vi "imagereg.vi"() -> ()   [LabVIEW 2012]
uses:
  <vilib>/Analysis/baseanly.llb/Mean (DBL).vi
  <vilib>/Analysis/NI_AALBase.lvlib
panel:
  in  "Tab":enum32{"Camera Init.", "Acquire"}(tab)
  in  "Constant\nfluor. amps":u16[](array[numeric])=[595, 455, 150, 360, 150]
  in  "Constant\npower amps":u16[](array[numeric])=[248, 455, 132, 266, 475]
  in  "DualView amps":u16[](array[numeric])=[1023, 760, 260, 800, 10]
  out "Initialize":u32
  out "Initialize?":bool
  out "x pixels":i32
  out "y pixels":i32
  out "Bits per Channel":i32
  out "Camera ID":string="0"
  out "Model":string="0"
  out "camera initialization error":errorcluster
  in  "Path":path
  in  "Contrast\nAdjust":cluster{i32, i32}(slide) scale=100.0..65535.0
  in  "Snap and save":bool
  out "Camera error":errorcluster caption="File error"
  in  "Enter live mode":bool
  in  "Exposure (msec)":dbl=100.0 min=1.0 max=5000.0 step=1.0
  out "Image":u16[][](graph)
  in  "stop program":bool
  out "File error":errorcluster
  in  "Red":bool
  in  "Yellow":bool
  in  "Orange":bool
  in  "Green":bool
  in  "Blue":bool
  in  "All":bool
  in  "RedP":bool
  in  "OrangeP":bool
  in  "GreenP":bool
  in  "YellowP":bool
  in  "BlueP":bool
  in  "rEff":dbl=0.99915395 format="%#_3g"
  in  "oEff":dbl=0.99914441 format="%#_3g"
  in  "yEff":dbl=0.99909989 format="%#_3g"
  in  "gEff":dbl=0.9990684 format="%#_3g"
  in  "bEff":dbl=0.99824746 format="%#_3g"
  in  "Emission filter":u16(ring)=2 items=["ET525/30"=7, "ET510LP"=1, "ET575/50"=2, "708/75"=3, "620LP"=4, "ET590/50M"=5, "HQ660LP"=6]
  out "mean":dbl=701.2764784557547
  out "max value":u16=1056
  out "min value":u16=384
  out "Histogram":T1(graph)={"X Values"=[417.6, 484.8, 552.0, 619.2, 686.4, 753.6, 820.8, 888.0, 955.2, 1022.4], "Histogram: h(x)"=[403, 4234, 6440, 8496, 9541, 10568, 10361, 4568, 669, 48]}
  in  "White Light Current (mA)":dbl=700.0
  in  "White LED":bool
  in  "Allow Manual Contrast Adj":bool
  in  "Clicky on Image":bool
  out "Output":dbl[][](array[numeric])
  # "Default AOTF settings (calibrated values are shown on the right)"
  # "595"
  # "455"
  # "150"
  # "360"
  # "150"
  # "248"
  # "455"
  # "132"
  # "266"
  # "475"
  # "700"
  # "760"
  # "260"
  # "800"
  # "40"
  # "Main Program"
  # "Live Controls"
  # "Shutter Control"
  # "AOTF Control"
  # "Laser Power Control"
  # "Measurements"
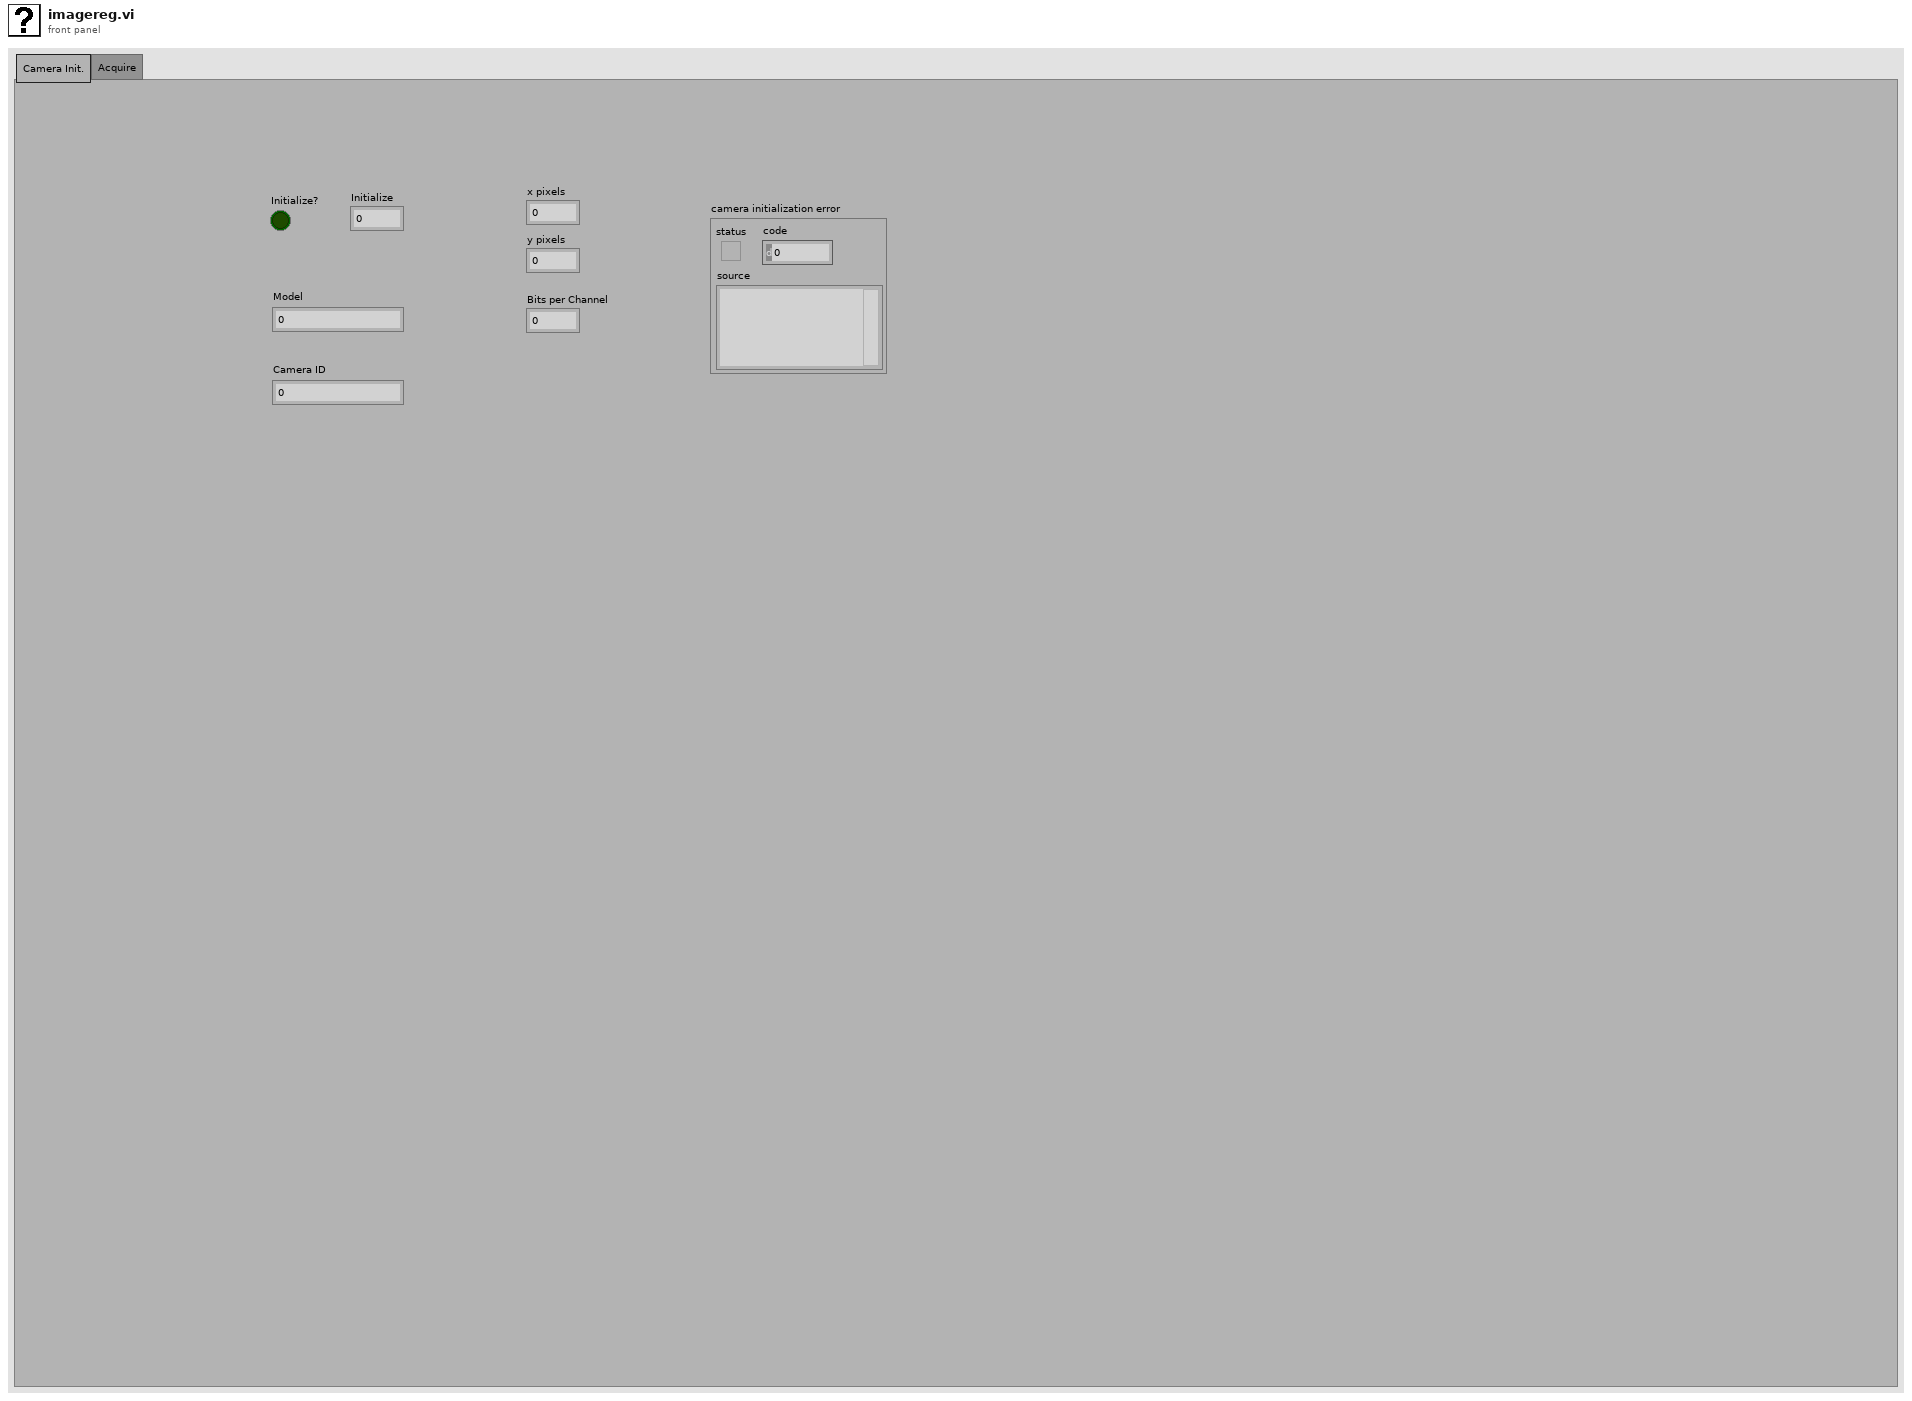
[diagram p1: front panel]
types:
  T1 = cluster{"X Values":dbl[], "Histogram: h(x)":i32[]}
  T2 = cluster{"Horizontal Offset":i32, "Vertical Offset":i32, "Horizontal Width":i32, "Vertical Width":i32}
  T3 = cluster{"Value":i32, "Minimum":i32, "Maximum":i32, "Increment":i32}
  T4 = cluster{"width":u32, "height":u32, "datatype":u32}
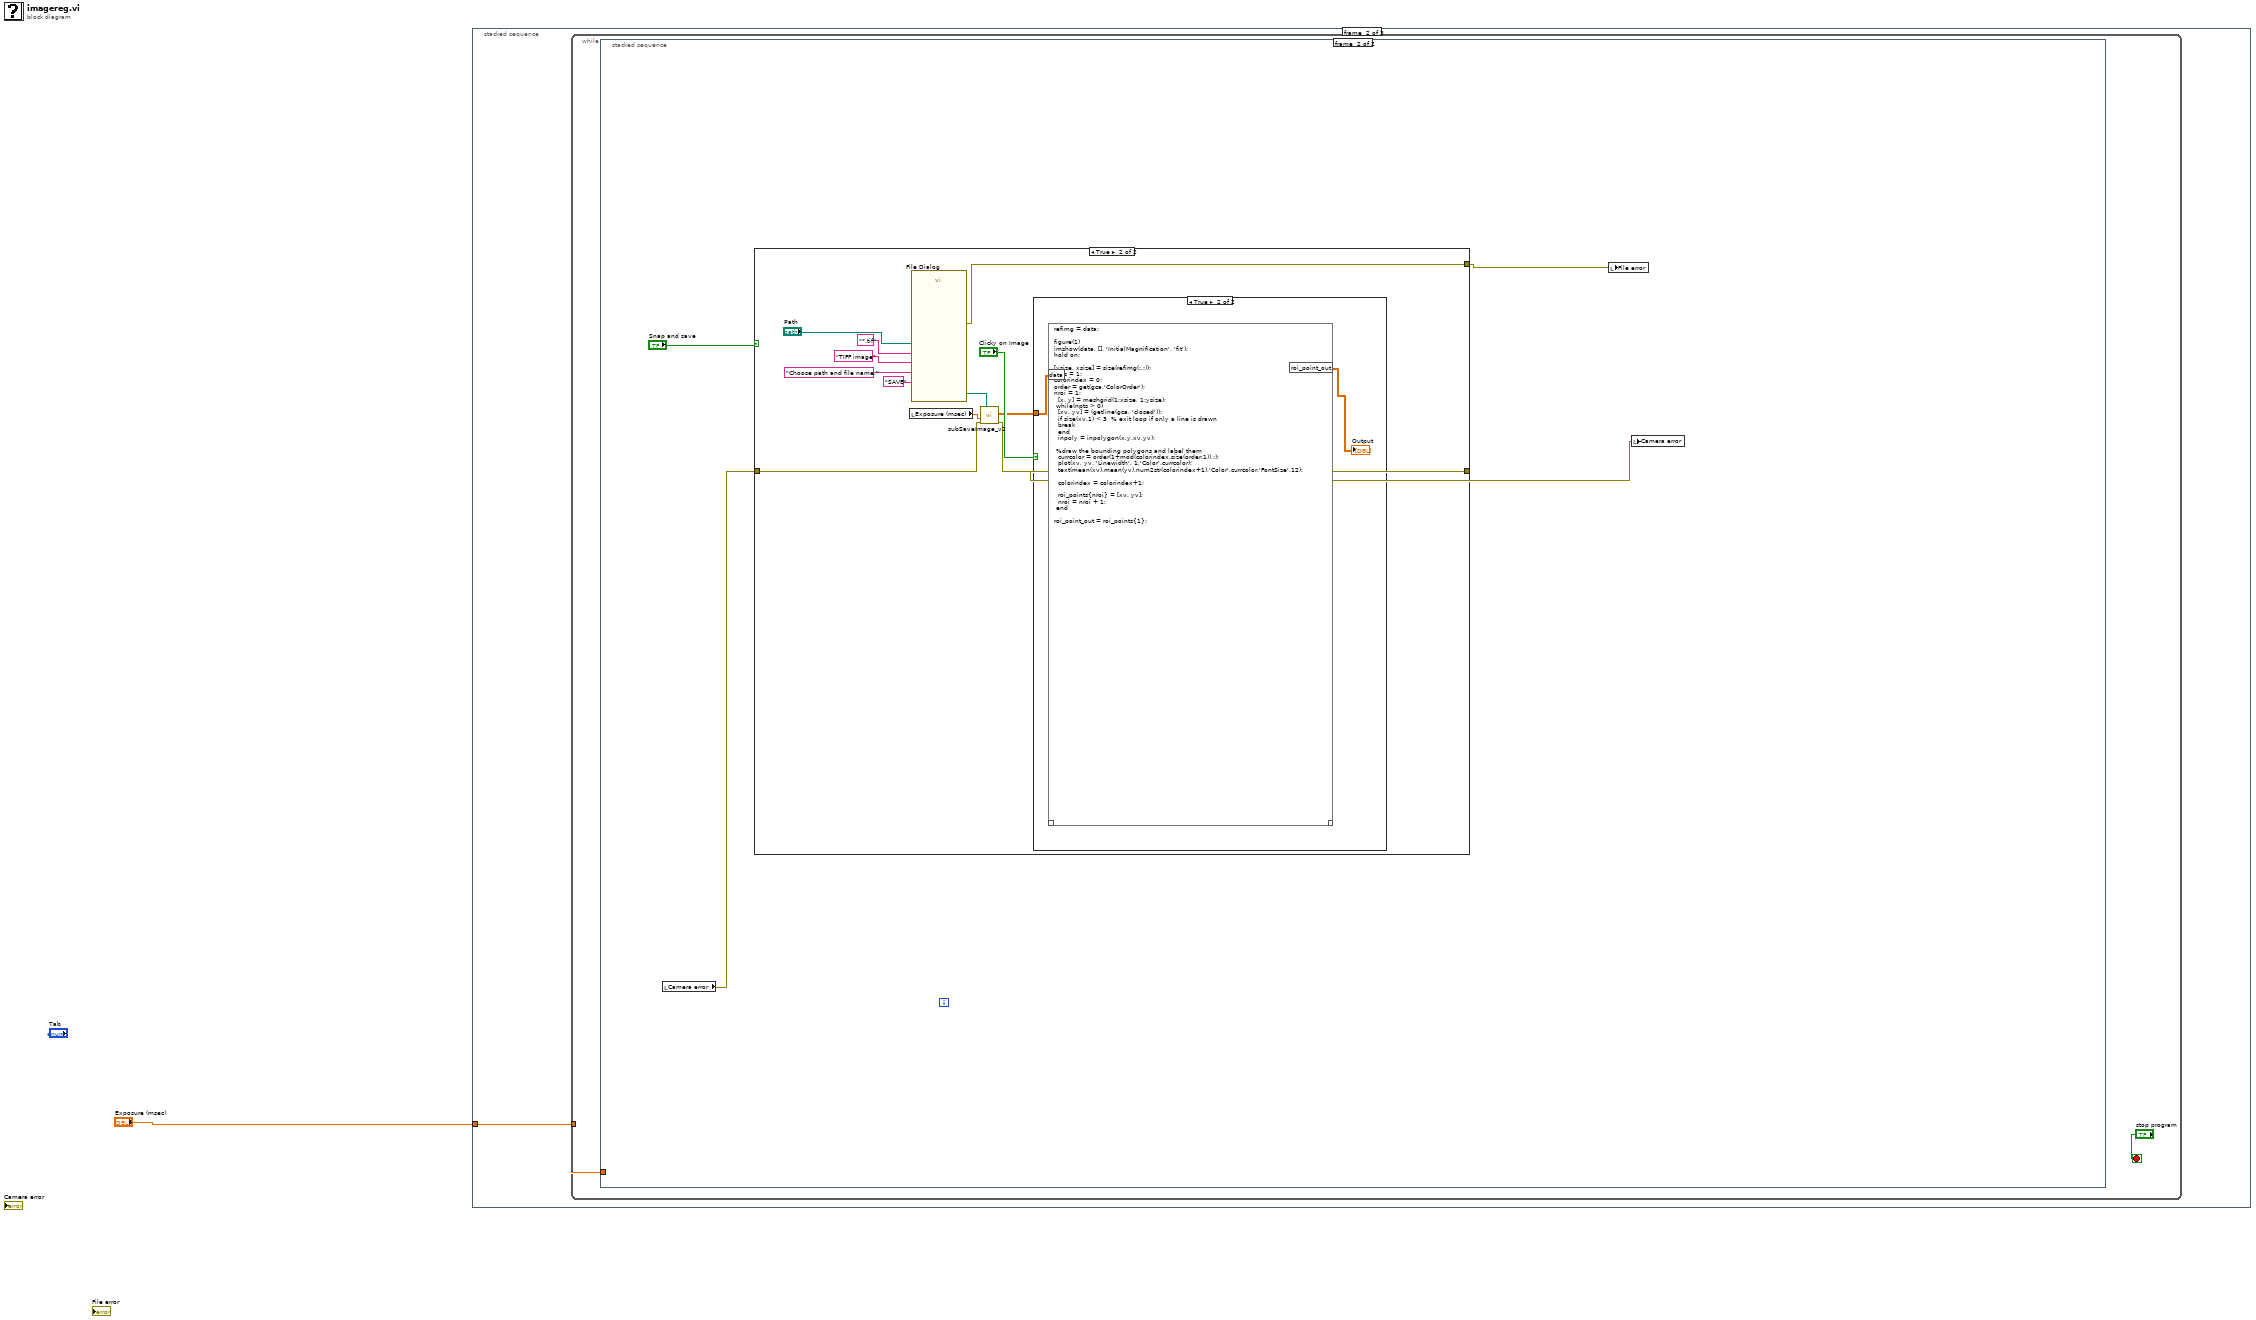
[diagram p0: block diagram]
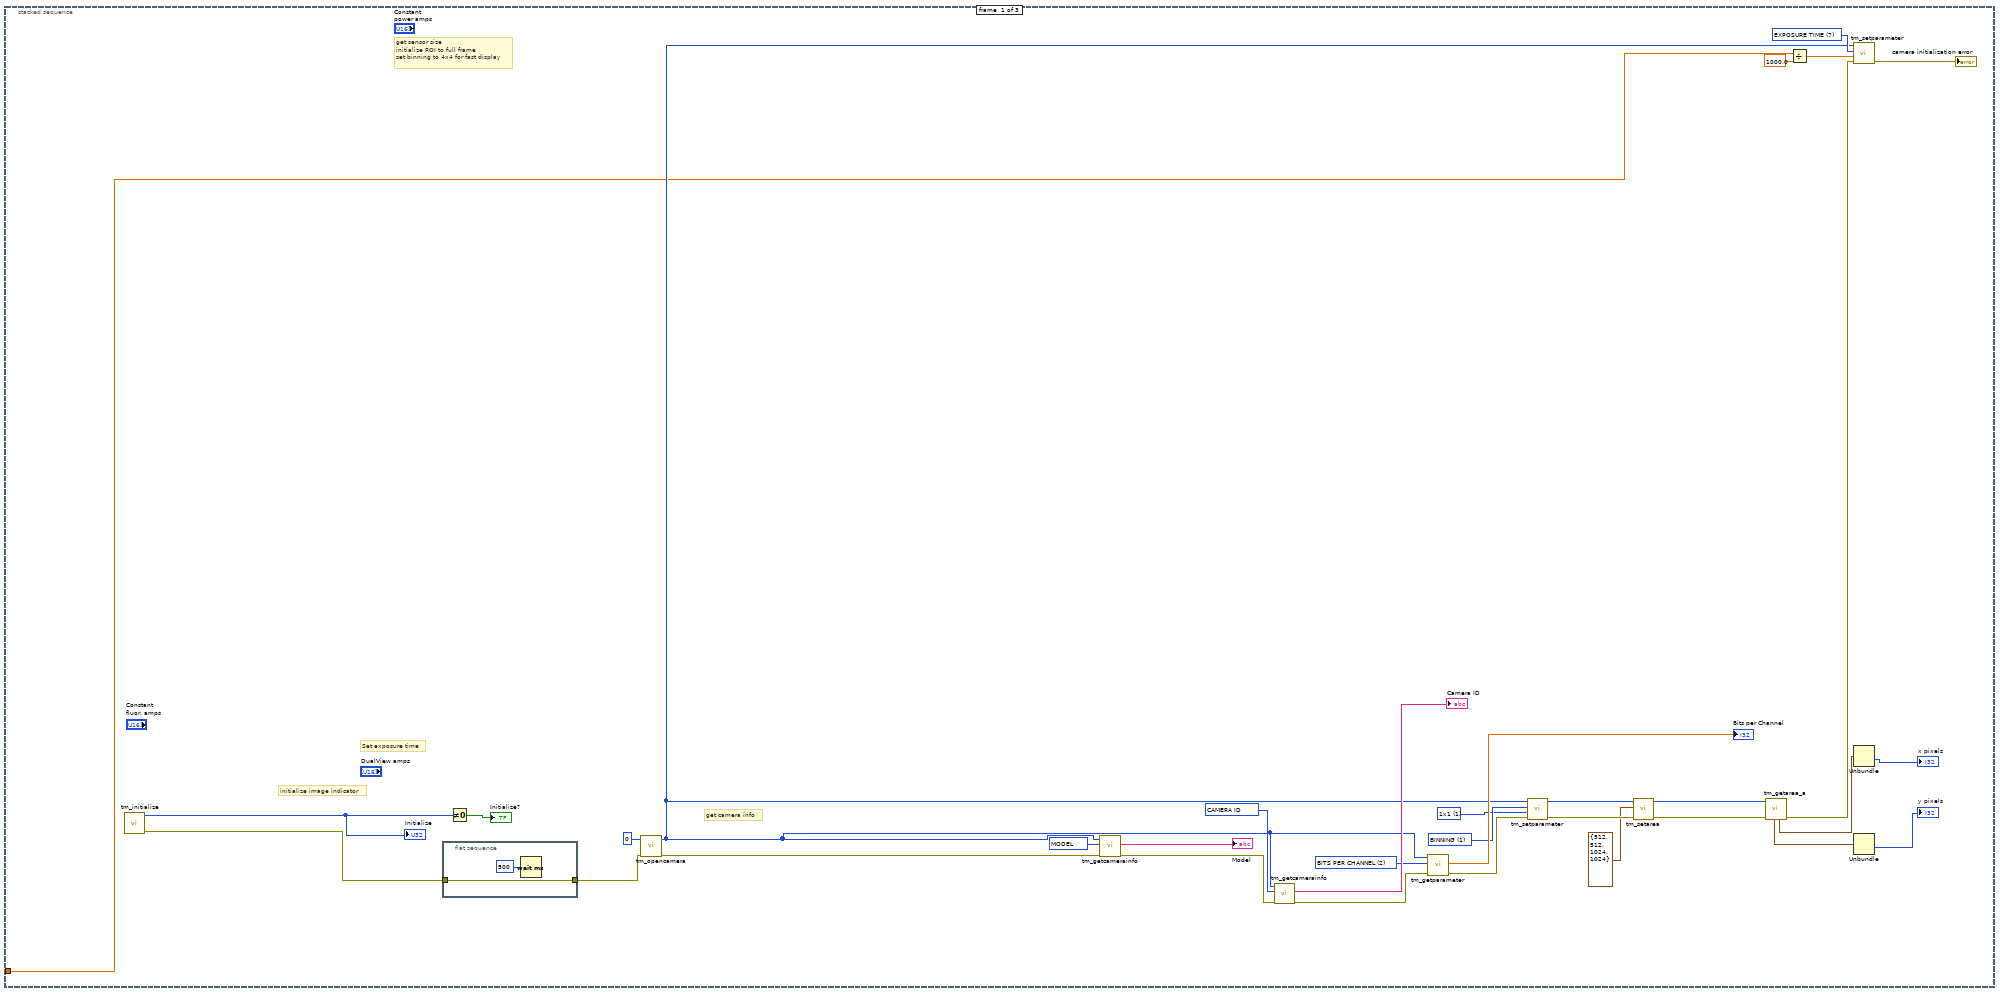
[diagram p2: hidden frame]
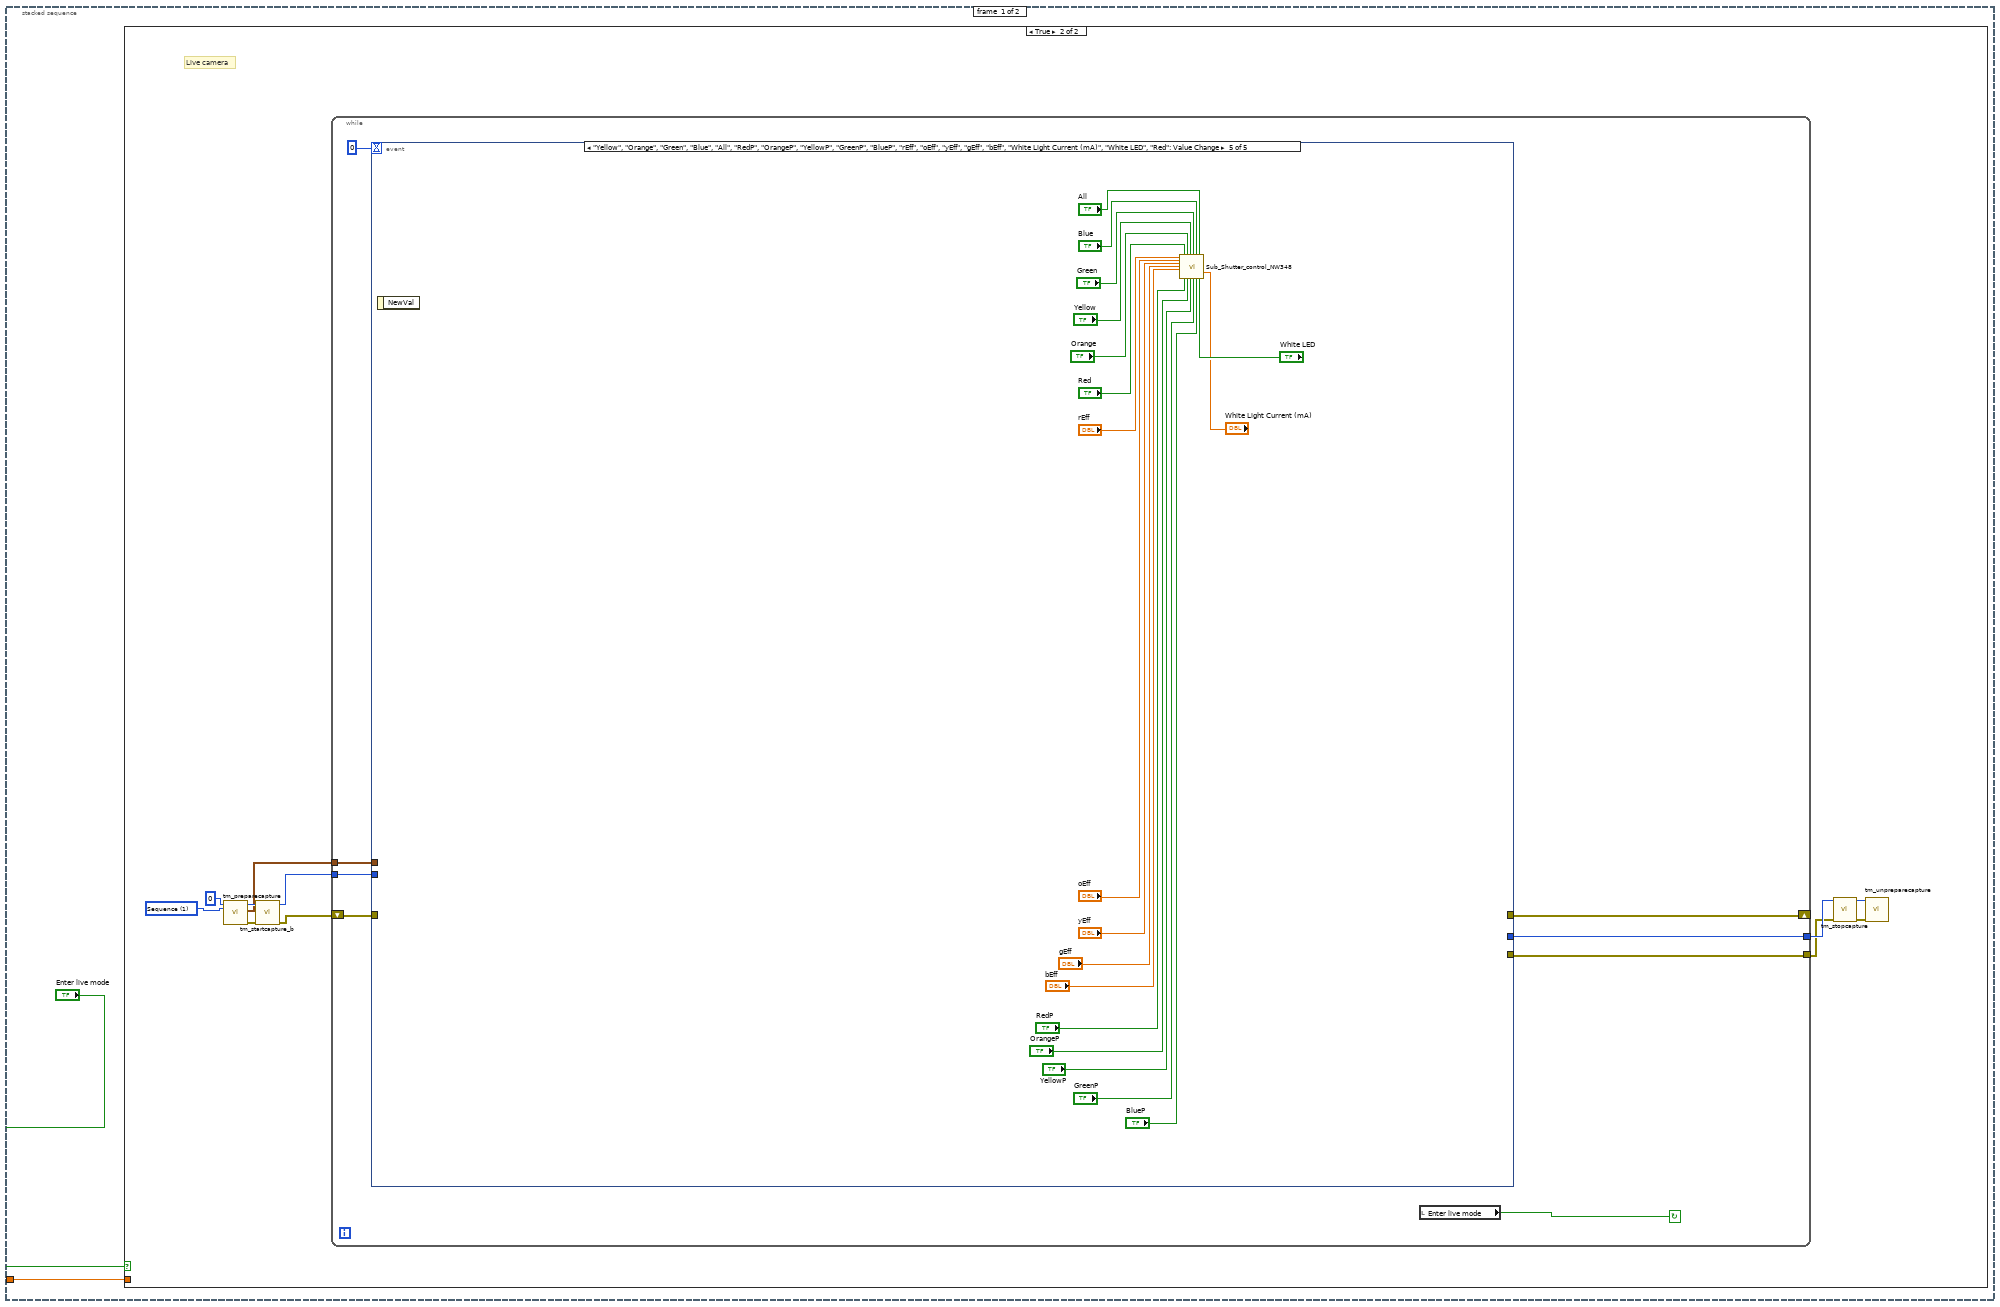
[diagram p3: hidden frame]
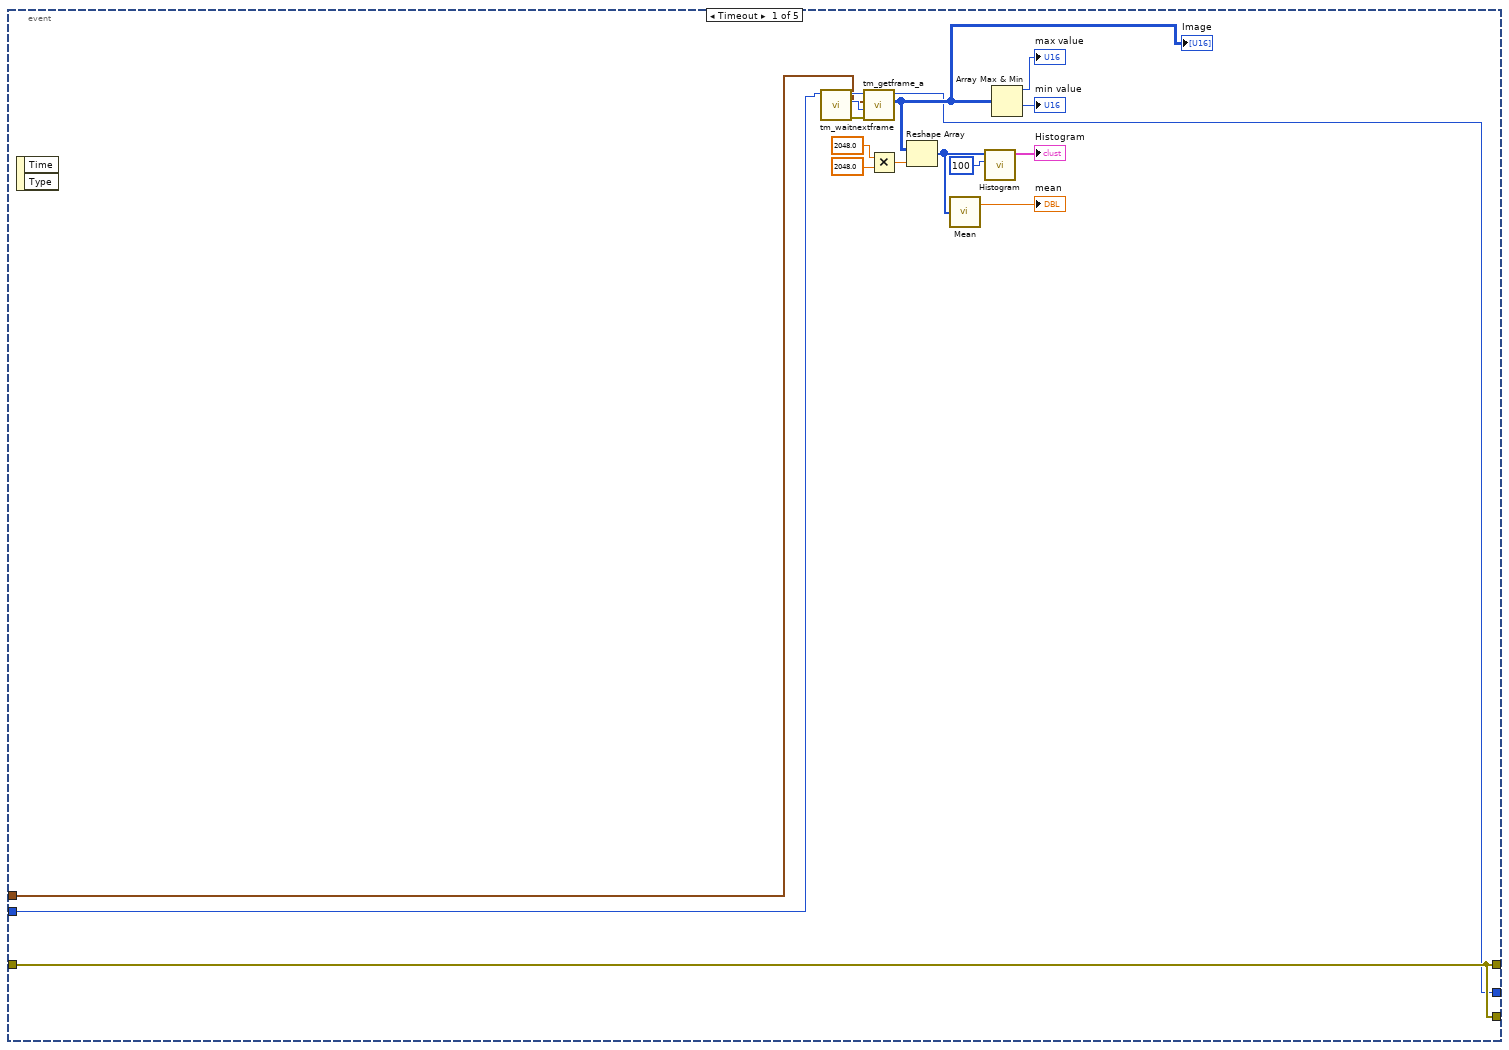
[diagram p5: hidden frame]
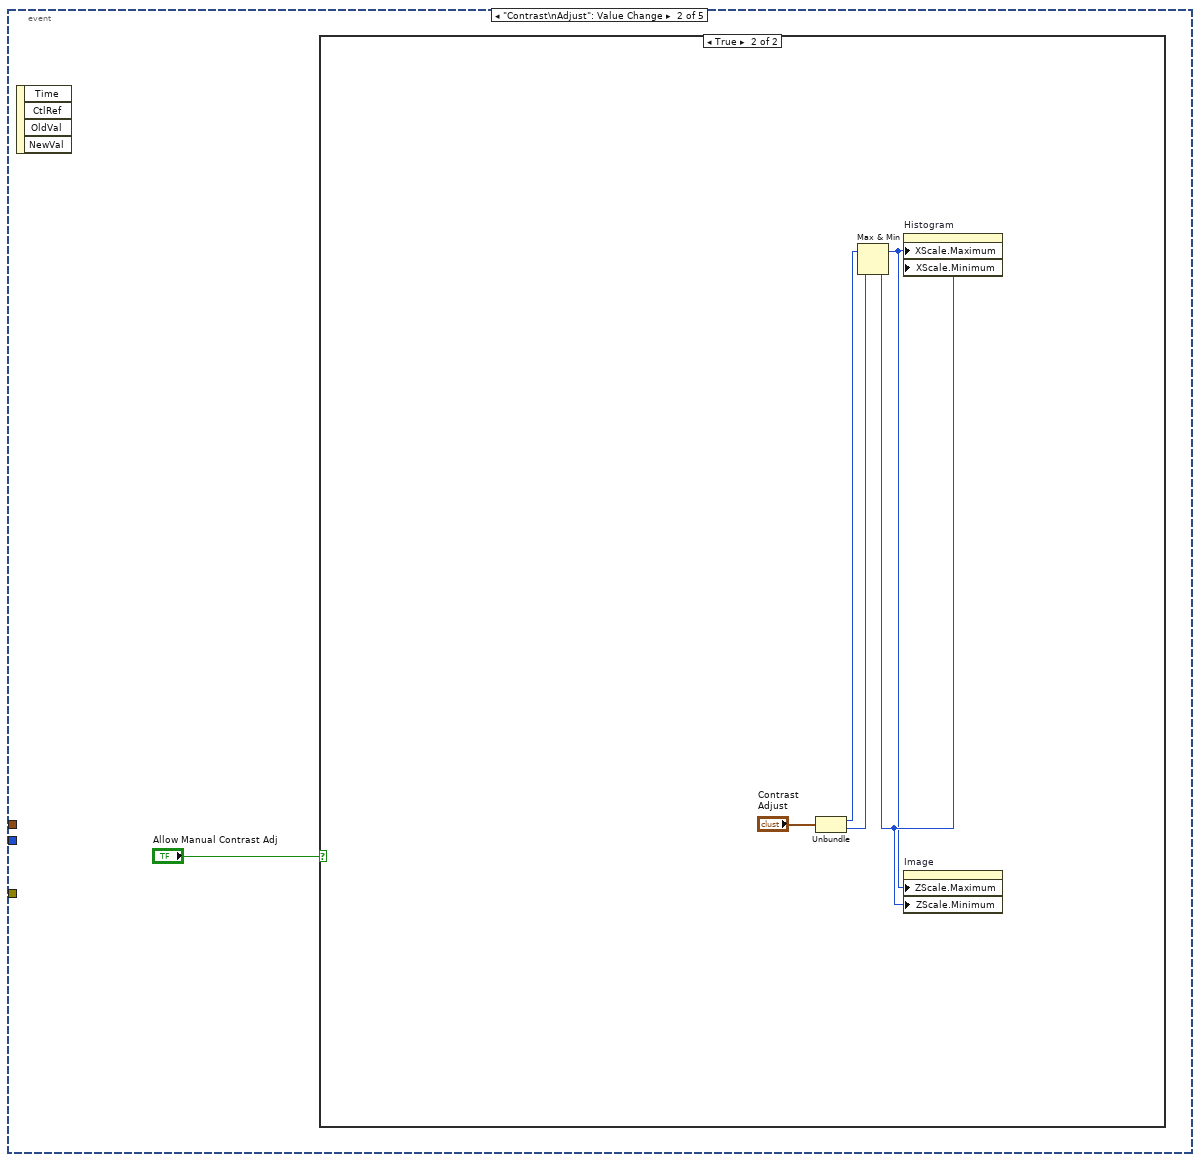
[diagram p6: hidden frame]
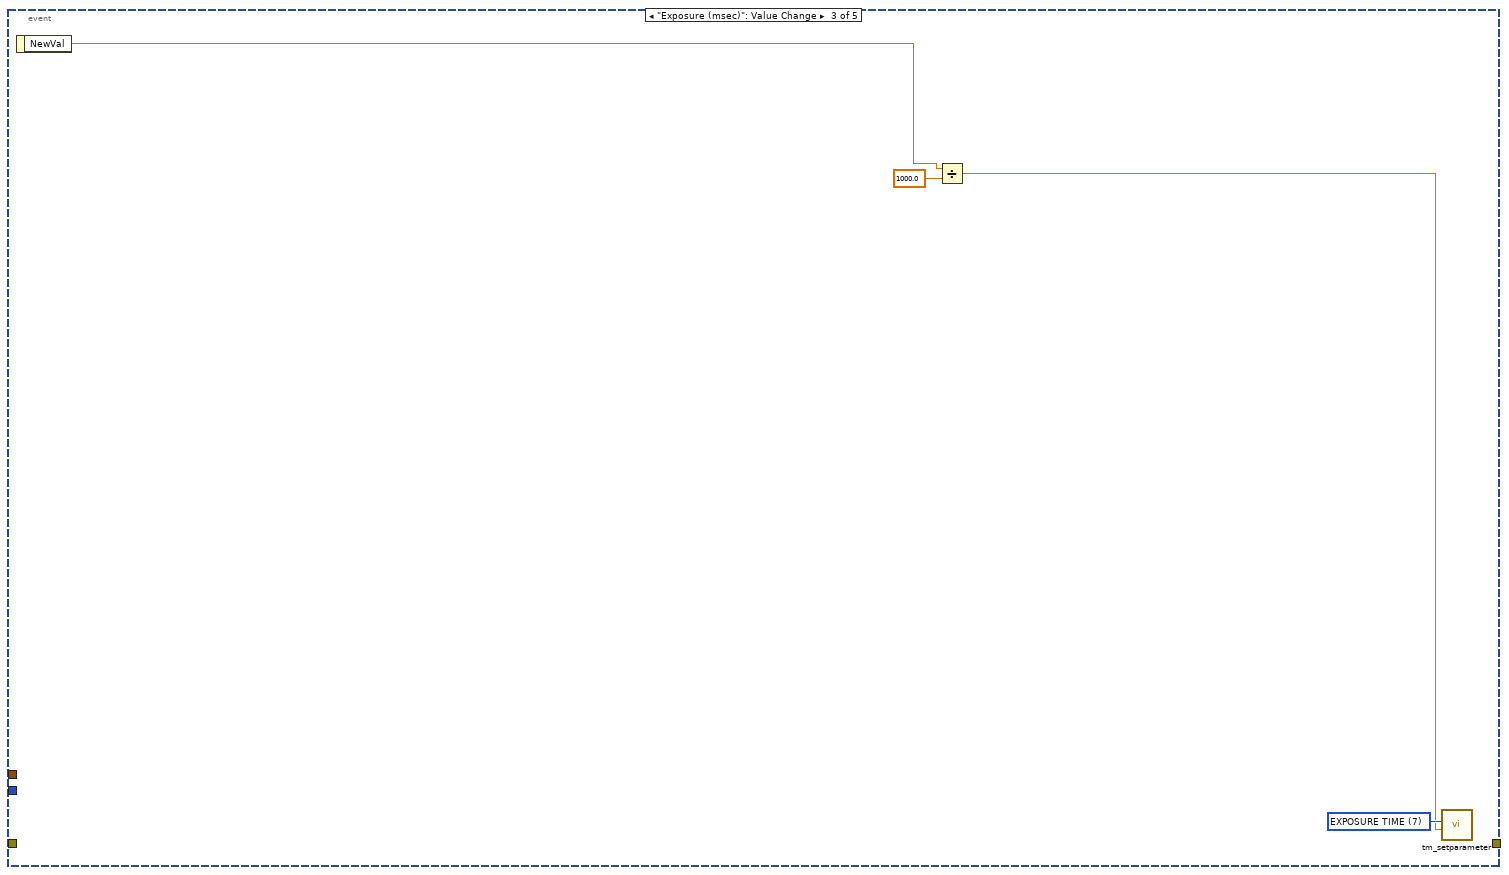
[diagram p8: hidden frame]
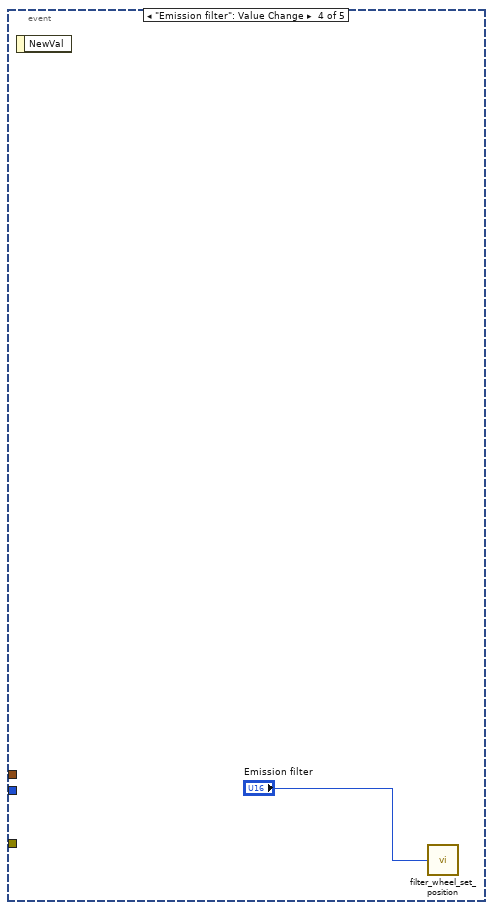
[diagram p9: hidden frame]
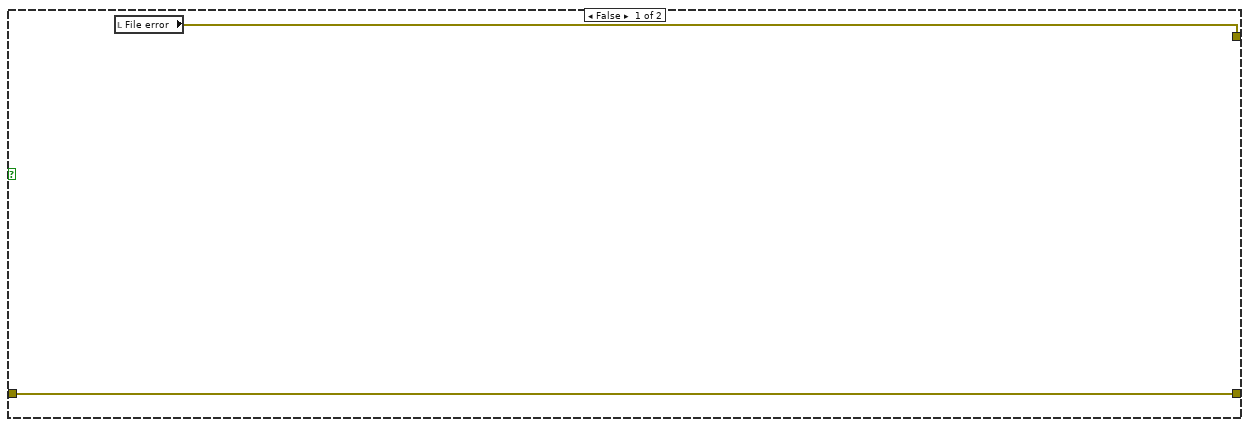
[diagram p10: hidden frame]
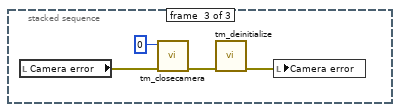
[diagram p12: hidden frame]
diagram:
  n1 = stacked-sequence {
    tunnel: "Exposure (msec)" -> [w10 w37 _]
    frame #0 {
      w9 = u16 1 items=["1x1"=1, "2x2"=2, "4x4"=4] ("Bin (n x n)")
      w16 = 7 items=["BINNING"=1, "BITS PER CHANNEL"=2, "ACTIVE VIEW INDEX"=3, "CCD MODE"=4, "SENSOR MODE"=5, "READOUT MODE"=6, "EXPOSURE TIME"=7, "CONTRAST GAIN"=8, "CONTRAST OFFSET"=9, "LIGHT MODE"=10, "SENSITIVITY"=11, "WHITE BALANCE"=12, "PHOTON IMAGING MODE"=13, "HIGH DYNAMIC RANGE MODE"=14, "TRIGGER SOURCE"=15, "TRIGGER ACTIVE"=16, "TRIGGER MODE"=17, "TRIGGER POLARITY"=18, "TRIGGER GLOBAL EXPOSURE"=19, "FIRST TRIGGER BEHAVIOR"=20, "TRIGGER TIMES"=21, "OUTPUT TRIGGER POLARITY"=22, "OUTPUT TRIGGER DELAY"=23, "OUTPUT TRIGGER PERIOD"=24, "TEMPERATURE"=25, "TEMPERATURE TARGET"=26, "SENSOR COOLER FAN"=27, "MECHANICAL SHUTTER"=28, "BACK FOCUS POSITION"=29, "FRAMEBUNDLE MODE"=30, "FRAMEBUNDLE NUMBER"=31, "LINEBUNDLE HEIGHT"=32, "TRIGGER CONNECTOR"=33, "IMAGE PIXEL TYPE"=34] ("Parameter")
      w20 = 1 items=["BINNING"=1, "BITS PER CHANNEL"=2, "ACTIVE VIEW INDEX"=3, "CCD MODE"=4, "SENSOR MODE"=5, "READOUT MODE"=6, "EXPOSURE TIME"=7, "CONTRAST GAIN"=8, "CONTRAST OFFSET"=9, "LIGHT MODE"=10, "SENSITIVITY"=11, "WHITE BALANCE"=12, "PHOTON IMAGING MODE"=13, "HIGH DYNAMIC RANGE MODE"=14, "TRIGGER SOURCE"=15, "TRIGGER ACTIVE"=16, "TRIGGER MODE"=17, "TRIGGER POLARITY"=18, "TRIGGER GLOBAL EXPOSURE"=19, "FIRST TRIGGER BEHAVIOR"=20, "TRIGGER TIMES"=21, "OUTPUT TRIGGER POLARITY"=22, "OUTPUT TRIGGER DELAY"=23, "OUTPUT TRIGGER PERIOD"=24, "TEMPERATURE"=25, "TEMPERATURE TARGET"=26, "SENSOR COOLER FAN"=27, "MECHANICAL SHUTTER"=28, "BACK FOCUS POSITION"=29, "FRAMEBUNDLE MODE"=30, "FRAMEBUNDLE NUMBER"=31, "LINEBUNDLE HEIGHT"=32, "TRIGGER CONNECTOR"=33, "IMAGE PIXEL TYPE"=34] ("Parameter")
      w22 = 2 items=["BINNING"=1, "BITS PER CHANNEL"=2, "ACTIVE VIEW INDEX"=3, "CCD MODE"=4, "SENSOR MODE"=5, "READOUT MODE"=6, "EXPOSURE TIME"=7, "CONTRAST GAIN"=8, "CONTRAST OFFSET"=9, "LIGHT MODE"=10, "SENSITIVITY"=11, "WHITE BALANCE"=12, "PHOTON IMAGING MODE"=13, "HIGH DYNAMIC RANGE MODE"=14, "TRIGGER SOURCE"=15, "TRIGGER ACTIVE"=16, "TRIGGER MODE"=17, "TRIGGER POLARITY"=18, "TRIGGER GLOBAL EXPOSURE"=19, "FIRST TRIGGER BEHAVIOR"=20, "TRIGGER TIMES"=21, "OUTPUT TRIGGER POLARITY"=22, "OUTPUT TRIGGER DELAY"=23, "OUTPUT TRIGGER PERIOD"=24, "TEMPERATURE"=25, "TEMPERATURE TARGET"=26, "SENSOR COOLER FAN"=27, "MECHANICAL SHUTTER"=28, "BACK FOCUS POSITION"=29, "FRAMEBUNDLE MODE"=30, "FRAMEBUNDLE NUMBER"=31, "LINEBUNDLE HEIGHT"=32, "TRIGGER CONNECTOR"=33, "IMAGE PIXEL TYPE"=34] ("Parameter")
      w28 = u32 67109122 items=["BUS"=67109121, "CAMERA ID"=67109122, "VENDOR"=67109123, "MODEL"=67109124, "CAMERA VERSION"=67109125, "DRIVER VERSION"=67109126, "MODULE VERSIOIN"=67109127, "DCAMAPI VERSION"=67109128] ("Info ID")
      w27 = u32 67109124 items=["BUS"=67109121, "CAMERA ID"=67109122, "VENDOR"=67109123, "MODEL"=67109124, "CAMERA VERSION"=67109125, "DRIVER VERSION"=67109126, "MODULE VERSIOIN"=67109127, "DCAMAPI VERSION"=67109128] ("Info ID")
      # "Set exposure time"
      # "initialize image indicator"
      # "get sensor size\ninitialize ROI to full frame\nset binning to 4x4 for fast display"
      # "get camera info"
      n2 = call <userlib>:"tm_initialize.vi"() -> ("error out"=w19:errorcluster, "Number Of Cameras"=w32:u32)  [unwired: 10 in]
      "Initialize" <- w32
      n3 = flat-sequence {
        tunnel: w19 -> [w35]
        tunnel: [w35] -> w18
        frame #0 {
          n4 = Wait (ms)(milliseconds to wait=u32 500) -> ()  [unwired: 1 out]
        }
      }
      n5 = Not Equal To 0?(x=w32) -> (x != 0?=→"Initialize?":bool)
      n6 = call <userlib>:"tm_opencamera.vi"("error in (no error)"=w18, "Camera Index"=u32 0 ("milliseconds to wait")) -> ("error out"=w30:errorcluster, "Handle out"=w15:u32)  [unwired: 8 in]
      n7 = call <userlib>:"tm_getcamerainfo.vi"("error in (no error)"=w30, "Info ID"=w27, "Handle in"=w15) -> ("error out"=w26:errorcluster, "String"=→"Model":string)  [unwired: 6 in, 1 out]
      n8 = call <userlib>:"tm_getcamerainfo.vi"("error in (no error)"=w26, "Info ID"=w28, "Handle in"=w15) -> ("error out"=w11:errorcluster, "String"=→"Camera ID":string)  [unwired: 6 in, 1 out]
      n9 = call <userlib>:"tm_getparameter.vi"("error in (no error)"=w11, "Parameter"=w22, "Handle in"=w15) -> ("error out"=w14:errorcluster, "Value out"=→"Bits per Channel":dbl)  [unwired: 6 in, 1 out]
      n10 = call <userlib>:"tm_setparameter.vi"("error in (no error)"=w14, "Value in"=w9, "Parameter"=w20, "Handle in"=w15) -> ("error out"=w4:errorcluster, "Handle out"=w6:u32)  [unwired: 6 in]
      n11 = call <userlib>:"tm_setarea.vi"("error in (no error)"=w4, "Sub Region"=T2 {"Horizontal Offset"=512, "Vertical Offset"=512, "Horizontal Width"=1024, "Vertical Width"=1024}, "Handle in"=w6) -> ("error out"=w3:errorcluster, "Handle out"=w5:u32)  [unwired: 7 in]
      n12 = call <userlib>:"tm_getarea_a.vi"("error in (no error)"=w3, "Handle in"=w5) -> ("error out"=w17:errorcluster, "H Width"=w24:T3, "V Width"=w23:T3)  [unwired: 4 in, 3 out]
      n13 = Divide(x=w10, y=1000.0) -> (x/y=w33:dbl)
      n14 = call <userlib>:"tm_setparameter.vi"("error in (no error)"=w17, "Value in"=w33, "Parameter"=w16, "Handle in"=w15) -> ("error out"=→"camera initialization error":errorcluster)  [unwired: 6 in, 1 out]
      n15 = Unbundle(w24) -> ("Maximum"=→"x pixels":i32)  [unwired: 3 out]
      n16 = Unbundle(w23) -> ("Maximum"=→"y pixels":i32)  [unwired: 3 out]
    }
    frame #1 {
      n17 = while {
        tunnel: w37 -> [w39]
        stop <- "stop program" stop-if-true
        n18 = stacked-sequence {
          tunnel: w39 -> [w41 _]
          frame #0 {
            n19 = case shown="True" "Enter live mode" {
              tunnel: w41 -> [_ _]
              frame False {
              }
              frame True {
                w47 = 1 items=["Snap", "Sequence"] ("Capture mode")
                # "Live camera"
                n20 = call <userlib>:"tm_preparecapture.vi"("Capture mode"=w47, "Handle in"=u32 0) -> ("error out"=w46:errorcluster, "Buffer"=w42:T4, "Handle out"=w45:u32)  [unwired: 6 in, 1 out]
                n21 = call <userlib>:"tm_startcapture_b.vi"("error in (no error)"=w46, "Handle in"=w45) -> ("error out"=w44:errorcluster, "Handle out"=w43:u32)  [unwired: 8 in]
                n22 = while {
                  shift-right: [w58] -> _
                  shift-left: w44 -> [w59]
                  tunnel: [w57] -> w52
                  tunnel: [w56] -> w51
                  tunnel: w43 -> [w55]
                  tunnel: w42 -> [w54]
                  stop <- w53 continue-if-true
                  n23 = event shown="[4] \"Yellow\", \"Orange\", \"Green\", \"Blue\", \"All\", \"RedP\", \"OrangeP\", \"YellowP\", \"GreenP\", \"BlueP\", \"rEff\", \"oEff\", \"yEff\", \"gEff\", \"bEff\", \"White Light Current (mA)\", \"White LED\", \"Red\": Value Change" {
                    selector: _ -> [_ _ _ _ _]
                    dyn-events: _ -> [_ _ _ _ _]
                    timeout: 0 -> [_ _ _ _ _]
                    tunnel: w59 -> [w65 _ _ _ _]
                    tunnel: [w65 _ _ _ _] -> w58
                    tunnel: [w61 _ _ _ _] -> w57
                    tunnel: [w65 _ _ _ _] -> w56
                    tunnel: w55 -> [w64 _ _ _ _]
                    tunnel: w54 -> [w62 _ _ _ _]
                    event Timeout {
                      n24 = event-data() -> ()  [unwired: 1 in, 2 out]
                      n25 = call <userlib>:"tm_waitnextframe.vi"("Handle in"=w64) -> ("error out"=w69:errorcluster, "Frame Index"=w71:i32, "Handle out"=w70:u32)  [unwired: 7 in, 1 out]
                      n26 = call <userlib>:"tm_getframe_a.vi"("error in (no error)"=w69, "Frame Index"=w71, "Buffer"=w62, "Handle in"=w70) -> ("Data 16"=w63:u16[][], "Handle out"=w61:u32)  [unwired: 4 in, 2 out]
                      "Image" <- w63
                      n27 = Multiply(x=2048.0, y=2048.0) -> (x*y=w75:dbl)
                      n28 = Reshape Array(w63, w75) -> (w77:u16[])
                      n29 = call-poly <vilib>:"Mean.vi"("X"=w77) -> ("mean"=→"mean":dbl)  [unwired: 1 out]
                      n30 = call <vilib>:"Histogram.vi"("intervals"=100, "X"=w77) -> ("Histogram Graph"=→"Histogram":T1)  [unwired: 6 in, 3 out]
                      n31 = Array Max & Min(array=w63) -> (max value=→"max value":u16, min value=→"min value":u16)  [unwired: 2 out]
                    }
                    event "Contrast\nAdjust": Value Change {
                      n32 = event-data() -> ()  [unwired: 1 in, 4 out]
                      n33 = case shown="True" "Allow Manual Contrast Adj" {
                        frame False {
                        }
                        frame True {
                          n34 = Unbundle("Contrast\nAdjust") -> (w82:i32, w83:i32)
                          n35 = Max & Min(x=w82, y=w83) -> (max(x,y)=w79:i32, min(x,y)=w80:i32)
                          n36 = property on="Histogram" class="XYGraph (strict)"("XScale.Maximum"=w79, "XScale.Minimum"=w80) -> ()  [unwired: 2 in, 2 out]
                          n37 = property on="Image" class="IntGraph (strict)"("ZScale.Maximum"=w79, "ZScale.Minimum"=w80) -> ()  [unwired: 2 in, 2 out]
                        }
                      }
                    }
                    event "Exposure (msec)": Value Change {
                      w87 = 7 items=["BINNING"=1, "BITS PER CHANNEL"=2, "ACTIVE VIEW INDEX"=3, "CCD MODE"=4, "SENSOR MODE"=5, "READOUT MODE"=6, "EXPOSURE TIME"=7, "CONTRAST GAIN"=8, "CONTRAST OFFSET"=9, "LIGHT MODE"=10, "SENSITIVITY"=11, "WHITE BALANCE"=12, "PHOTON IMAGING MODE"=13, "HIGH DYNAMIC RANGE MODE"=14, "TRIGGER SOURCE"=15, "TRIGGER ACTIVE"=16, "TRIGGER MODE"=17, "TRIGGER POLARITY"=18, "TRIGGER GLOBAL EXPOSURE"=19, "FIRST TRIGGER BEHAVIOR"=20, "TRIGGER TIMES"=21, "OUTPUT TRIGGER POLARITY"=22, "OUTPUT TRIGGER DELAY"=23, "OUTPUT TRIGGER PERIOD"=24, "TEMPERATURE"=25, "TEMPERATURE TARGET"=26, "SENSOR COOLER FAN"=27, "MECHANICAL SHUTTER"=28, "BACK FOCUS POSITION"=29, "FRAMEBUNDLE MODE"=30, "FRAMEBUNDLE NUMBER"=31, "LINEBUNDLE HEIGHT"=32, "TRIGGER CONNECTOR"=33, "IMAGE PIXEL TYPE"=34] ("Parameter")
                      n38 = event-data() -> ("NewVal"=w85:dbl)  [unwired: 1 in]
                      n39 = Divide(x=w85, y=1000.0) -> (x/y=w84:dbl)
                      n40 = call <userlib>:"tm_setparameter.vi"("Value in"=w84, "Parameter"=w87) -> ()  [unwired: 8 in, 2 out]
                    }
                    event "Emission filter": Value Change {
                      n41 = event-data() -> ()  [unwired: 1 in, 1 out]
                      n42 = call "filter_wheel_set_position.vi"("Filter Wheel Position - Control"="Emission filter") -> ()
                    }
                    event "Yellow", "Orange", "Green", "Blue", "All", "RedP", "OrangeP", "YellowP", "GreenP", "BlueP", "rEff", "oEff", "yEff", "gEff", "bEff", "White Light Current (mA)", "White LED", "Red": Value Change {
                      n43 = event-data() -> ()  [unwired: 1 in, 1 out]
                      n44 = call "Sub_Shutter_control_NW348.vi"("rEff"="rEff", "oEff"="oEff", "yEff"="yEff", "gEff"="gEff", "bEff"="bEff", "White Light Current (mA)"="White Light Current (mA)", "Red"="Red", "RedP"="RedP", "Orange"="Orange", "OrangeP"="OrangeP", "Yellow"="Yellow", "YellowP"="YellowP", "Green"="Green", "GreenP"="GreenP", "Blue"="Blue", "BlueP"="BlueP", "All"="All", "White LED"="White LED") -> ()  [unwired: 10 in]
                    }
                  }
                  n45 = local read "Enter live mode"() -> (w53:bool)
                }
                n46 = call <userlib>:"tm_stopcapture.vi"("error in (no error)"=w51, "Handle in"=w52) -> ("error out"=w49:errorcluster, "Handle out"=w50:u32)  [unwired: 8 in]
                n47 = call <userlib>:"tm_unpreparecapture.vi"("error in (no error)"=w49, "Handle in"=w50) -> ()  [unwired: 8 in, 2 out]
              }
            }
          }
          frame #1 {
            n48 = local read "Camera error"() -> (w110:errorcluster)
            n49 = case shown="True" "Snap and save" {
              tunnel: [w111 w120] -> w107
              tunnel: w110 -> [w112 w116]
              tunnel: [w112 w115] -> w108
              frame False {
                n50 = local read "File error"() -> (w111:errorcluster)
              }
              frame True {
                n51 = local read "Exposure (msec)"() -> (w117:dbl)
                n52 = call "File Dialog"("start path"="Path", "prompt"="Choose path and file name.", "button label"="SAVE", "pattern (all files)"="*.tif" ("default name"), "pattern label"="TIFF image" ("default name")) -> ("selected path"=w118:path, "error out"=w120:errorcluster)  [unwired: 7 in, 2 out]
                n53 = call "subSaveImage_v2.vi"("File name"=w118, "Camera error in"=w116, "Exposure (msec)"=w117) -> ("Camera error out"=w115:errorcluster, "Image Data"=w113:dbl[][])  [unwired: 7 in]
                n54 = case shown="True" "Clicky on Image" {
                  tunnel: w113 -> [_ w125]
                  frame False {
                  }
                  frame True {
                    n55 = script code="refimg = data;\n\nfigure(1)\nimshow(data, [], 'InitialMagnification', 'fit');\nhold on;\n\n[ysize, xsize] = size(refimg(:,:)); \nnpts = 1;\ncolorindex = 0;\norder = get(gca,'ColorOrder');\nnroi = 1;\n  [x, y] = meshgrid(1:xsize, 1:ysize);\n while(npts > 0)\n  [xv, yv] = (getline(gca, 'closed'));\n  if size(xv,1) < 3  % exit loop if only a line is drawn\n  break\n  end\n  inpoly = inpolygon(x,y,xv,yv);\n  \n %draw the bounding polygons and label them\n  currcolor = order(1+mod(colorindex,size(order,1)),:);\n  plot(xv, yv, 'Linewidth', 1,'Color',currcolor);\n  text(mean(xv),mean(yv),num2str(colorindex+1),'Color',currcolor,'FontSize',12);\n\n  colorindex = colorindex+1;\n \n  roi_points{nroi} = [xv, yv];\n  nroi = nroi + 1;\n end\n\nroi_point_out = roi_points{1};"("data"=w125) -> ("roi_point_out"=→"Output":dbl[][])  [unwired: 1 in, 1 out]
                  }
                }
              }
            }
            n56 = local write "File error"(w107) -> ()
            n57 = local write "Camera error"(w108) -> ()
          }
        }
      }
    }
    frame #2 {
      n58 = local read "Camera error"() -> (w127:errorcluster)
      n59 = call <userlib>:"tm_closecamera.vi"("error in (no error)"=w127, "Handle in"=u32 0) -> ("error out"=w129:errorcluster)  [unwired: 9 in]
      n60 = call <userlib>:"tm_deinitialize.vi"("error in (no error)"=w129) -> ("error out"=w130:errorcluster)  [unwired: 10 in]
      n61 = local write "Camera error"(w130) -> ()
    }
  }
